vi "Find Stat Bundle Indexes.vi"(5 "IDs":string[](array[string]), 9 "DeletedIndex":i32) -> (4 "StartIndex":i32, 8 "EndIndex":i32, 15 "DeleteStatSet":bool)   [LabVIEW 2013]
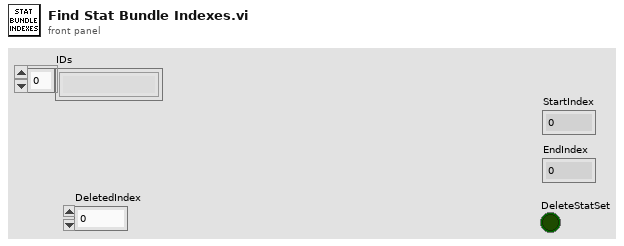
[diagram p1: front panel]
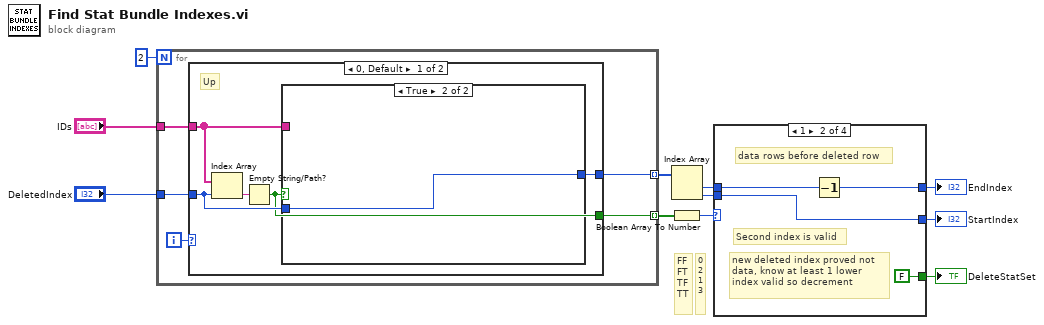
[diagram p0: block diagram]
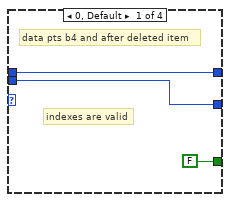
[diagram p2: hidden frame]
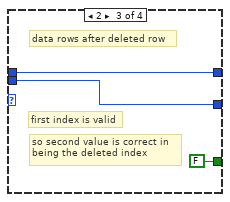
[diagram p3: hidden frame]
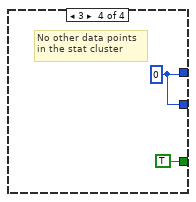
[diagram p4: hidden frame]
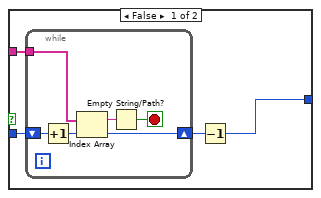
[diagram p5: hidden frame]
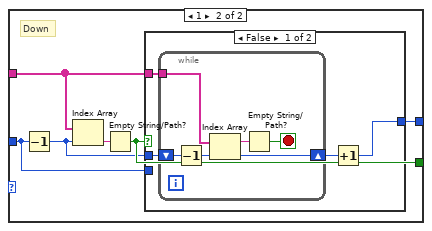
[diagram p6: hidden frame]
diagram:
  # "FF\nFT\nTF\nTT"
  # "0\n2\n1\n3"
  n1 = for {
    N: 2 -> [_]
    tunnel: "DeletedIndex" -> [w14]
    tunnel: "IDs" -> [w15]
    tunnel: [w13] -> w3 mode=indexing
    tunnel: [w12] -> w8 mode=indexing
    i -> [w16]
    n2 = case shown="0, Default" w16 {
      tunnel: w15 -> [w20 w36]
      tunnel: w14 -> [w19 w32]
      tunnel: [w18 w35] -> w12
      tunnel: [w17 w34] -> w13
      frame 0, Default {
        # "Up"
        n3 = Index Array(array=w20, index=w19) -> (element=w21:string)
        n4 = Empty String/Path?(string/path=w21) -> (empty?=w18:bool)
        n5 = case shown="True" w18 {
          tunnel: w20 -> [w24 _]
          tunnel: w19 -> [w25 w31]
          tunnel: [w22 w31] -> w17
          frame False {
            n6 = while {
              tunnel: w24 -> [w30]
              shift-right: [w28] -> w23
              shift-left: w25 -> [w29]
              stop <- w26 stop-if-true
              n7 = Increment(x=w29) -> (x+1=w28:i32)
              n8 = Index Array(array=w30, index=w28) -> (element=w27:string)
              n9 = Empty String/Path?(string/path=w27) -> (empty?=w26:bool)
            }
            n10 = Decrement(x=w23) -> (x-1=w22:i32)
          }
          frame True {
          }
        }
      }
      frame 1 {
        # "Down"
        n11 = Decrement(x=w32) -> (x-1=w33:i32)
        n12 = Index Array(array=w36, index=w33) -> (element=w37:string)
        n13 = Empty String/Path?(string/path=w37) -> (empty?=w35:bool)
        n14 = case shown="False" w35 {
          tunnel: w36 -> [w40 _]
          tunnel: w33 -> [w41 _]
          tunnel: [w38 w47] -> w34
          tunnel: w32 -> [_ w47]
          frame False {
            n15 = while {
              tunnel: w40 -> [w46]
              shift-right: [w44] -> w39
              shift-left: w41 -> [w45]
              stop <- w42 stop-if-true
              n16 = Decrement(x=w45) -> (x-1=w44:i32)
              n17 = Index Array(array=w46, index=w44) -> (element=w43:string)
              n18 = Empty String/Path?(string/path=w43) -> (empty?=w42:bool)
            }
            n19 = Increment(x=w39) -> (x+1=w38:i32)
          }
          frame True {
          }
        }
      }
    }
  }
  n20 = Index Array(array=w3) -> (element #1=w2:i32, element #2=w1:i32)  [unwired: 2 in]
  n21 = Boolean Array To Number(Boolean array=w8) -> (number=w7:u32)
  n22 = case shown="1" w7 {
    tunnel: [FALSE FALSE FALSE TRUE] -> w6
    tunnel: [w49 w51 w56 w58] -> w4
    tunnel: [w48 w53 w55 w58] -> w5
    tunnel: w2 -> [w49 w52 w56 _]
    tunnel: w1 -> [w48 w53 w55 _]
    frame 0, Default {
      # "indexes are valid"
      # "data pts b4 and after deleted item"
    }
    frame 1 {
      # "new deleted index proved not\ndata, know at least 1 lower\nindex valid so decrement"
      # "data rows before deleted row"
      # "Second index is valid"
      n23 = Decrement(x=w52) -> (x-1=w51:i32)
    }
    frame 2 {
      # "so second value is correct in\nbeing the deleted index"
      # "data rows after deleted row"
      # "first index is valid"
    }
    frame 3 {
      w58 = 0 ("DeletedIndex")
      # "No other data points\nin the stat cluster"
    }
  }
  "DeleteStatSet" <- w6
  "StartIndex" <- w5
  "EndIndex" <- w4
